vi "rs3 init post-process.vi"(8 "error in (no error)":errorcluster) -> (0 "error out":errorcluster, 2 "Processing Queues":T1, 3 "Processing Blocks":T2)   [LabVIEW 2018, in "libRealSense3.lvlib"]
doc: "This initializes the processing blocks and queues for the \n1. Subsampling\n2. Transform to disparity space\n3. Spatial filter\n4. Transform back to depth space\n5. Temporal filter"
uses:
  libRealSense3.lvlib
panel:
  # "RS3 Init Post-Process"
  # "(C) Intel Corp.,  AGJ"
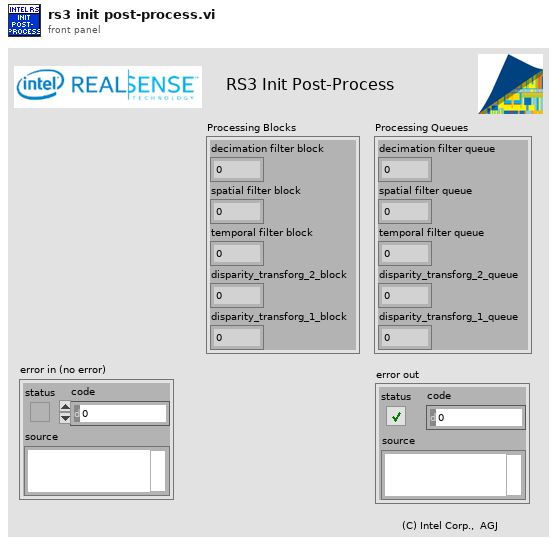
[diagram p1: front panel]
types:
  T1 = cluster{"decimation filter queue":u64, "spatial filter queue":u64, "temporal filter queue":u64, "disparity_transforg_2_queue":u64, "disparity_transforg_1_queue":u64}
  T2 = cluster{"decimation filter block":u64, "spatial filter block":u64, "temporal filter block":u64, "disparity_transforg_2_block":u64, "disparity_transforg_1_block":u64}
  T3 = cluster{"decimation filter queue":u64, "spatial filter queue":u64, "temporal filter queue":u64, "disparity transforg_2_queue":u64, "disparity transforg_1_queue":u64}
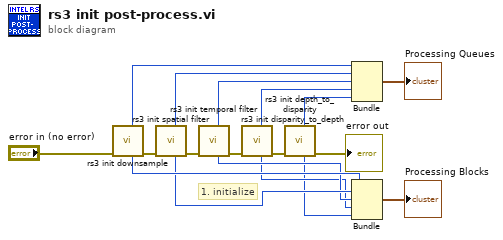
[diagram p0: block diagram]
diagram:
  # "1. initialize"
  n1 = call "rs3 init downsample.vi"("error in (no error)"="error in (no error)") -> ("error out"=w16:errorcluster, "decimation filter block"=w12:u64, "decimation filter queue"=w5:u64)  [unwired: 5 in, 3 out]
  n2 = call "rs3 init spatial filter.vi"("error in (no error)"=w16) -> ("error out"=w15:errorcluster, "spatial filter block"=w11:u64, "spatial filter queue"=w4:u64)  [unwired: 5 in, 3 out]
  n3 = call "rs3 init temporal filter.vi"("error in (no error)"=w15) -> ("error out"=w14:errorcluster, "temporal filter block"=w10:u64, "temporal filter queue"=w3:u64)  [unwired: 5 in, 3 out]
  n4 = call "rs3 init disparity_to_depth.vi"("error in (no error)"=w14) -> ("error out"=w13:errorcluster, "disparity_transforg_2_block"=w9:u64, "disparity transforg_2_queue"=w2:u64)  [unwired: 5 in, 3 out]
  n5 = call "rs3 init depth_to_disparity.vi"("error in (no error)"=w13) -> ("error out"=→"error out":errorcluster, "disparity_transforg_1_block"=w8:u64, "disparity transforg_1_queue"=w1:u64)  [unwired: 5 in, 3 out]
  n6 = Bundle("decimation filter queue"=w5, "spatial filter queue"=w4, "temporal filter queue"=w3, "disparity transforg_2_queue"=w2, "disparity transforg_1_queue"=w1) -> (→"Processing Queues":T3)  [unwired: 1 in]
  n7 = Bundle("decimation filter block"=w12, "spatial filter block"=w11, "temporal filter block"=w10, "disparity_transforg_2_block"=w9, "disparity_transforg_1_block"=w8) -> (→"Processing Blocks":T2)  [unwired: 1 in]
